vi "setPrevious.vi"(8 "error in (no error)":errorcluster, 10 "previous":refnum<data-value>, 11 "LLNode in":refnum<class "LLNode.lvclass">) -> (0 "error out":errorcluster, 3 "LLNode out":refnum<class "LLNode.lvclass">)   [LabVIEW 2009, in "LLNode.lvclass"]
doc: "Sets the Previous node in the linked list."
uses:
  LLNode.lvclass
  LLNode.lvclass/LLNode.ctl
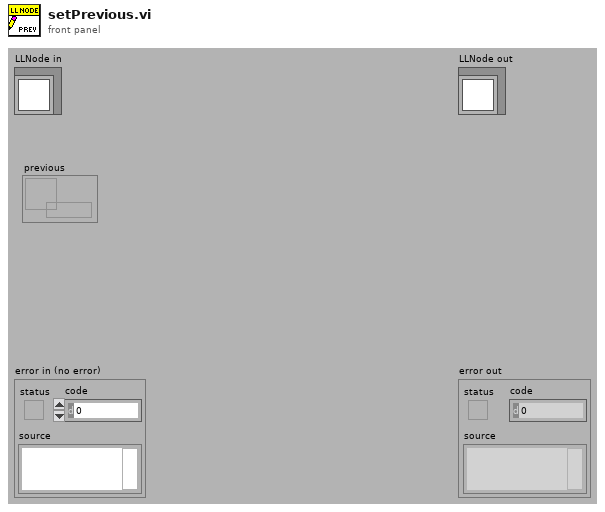
[diagram p1: front panel]
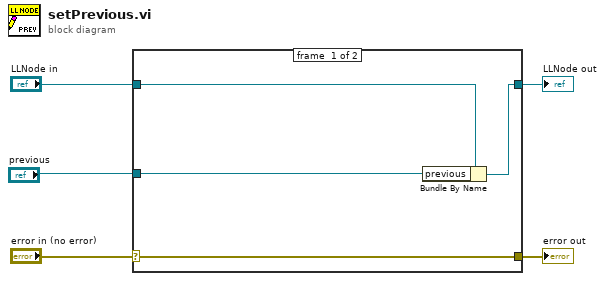
[diagram p0: block diagram]
diagram:
  n1 = case shown="No Error" "error in (no error)" {
    selector: "error in (no error)" -> [w9 w10]
    tunnel: [w9 w10] -> w4
    tunnel: [w7 w11] -> w2
    tunnel: "LLNode in" -> [w8 w11]
    tunnel: "previous" -> [w6 _]
    frame #0 {
      n2 = Bundle By Name(cluster=w8, "previous"=w6) -> (w7:refnum<class "LLNode.lvclass">)
    }
    frame #1 {
    }
  }
  "error out" <- w4
  "LLNode out" <- w2
